vi "provide_OME_data.vi"(6 "image ID":string, 8 "error in (no error)":errorcluster, 9 "structuredAttribute string in":string, 10 "OME element in":refnum<class "XMLElement.lvclass">, 11 "GenericDataCollection in":refnum<class "GenericDataCollection.lvclass">) -> (0 "error out":errorcluster, 1 "structuredAttribute string out":string, 2 "OME element out":refnum<class "XMLElement.lvclass">, 3 "GenericDataCollection out":refnum<class "GenericDataCollection.lvclass">)   [LabVIEW 2010, in "GenericDataCollection.lvclass"]
uses:
  GenericDataCollection.lvclass
  common/classes/XMLElement/XMLElement/XMLElement.lvclass
  ImagingMode/GenericImagingMode/GenericImagingMode/GenericImagingMode.lvclass
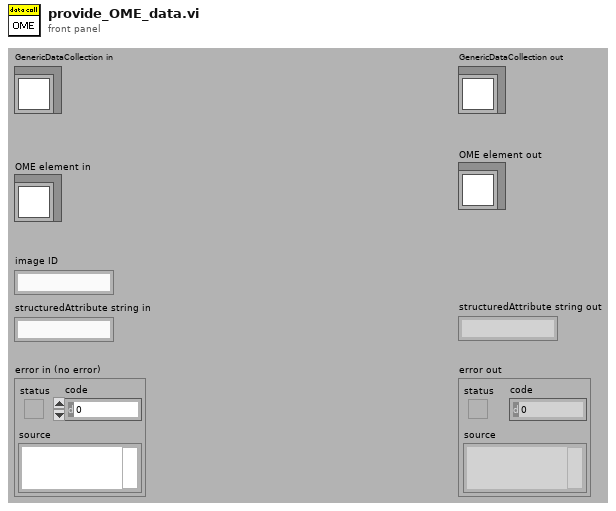
[diagram p1: front panel]
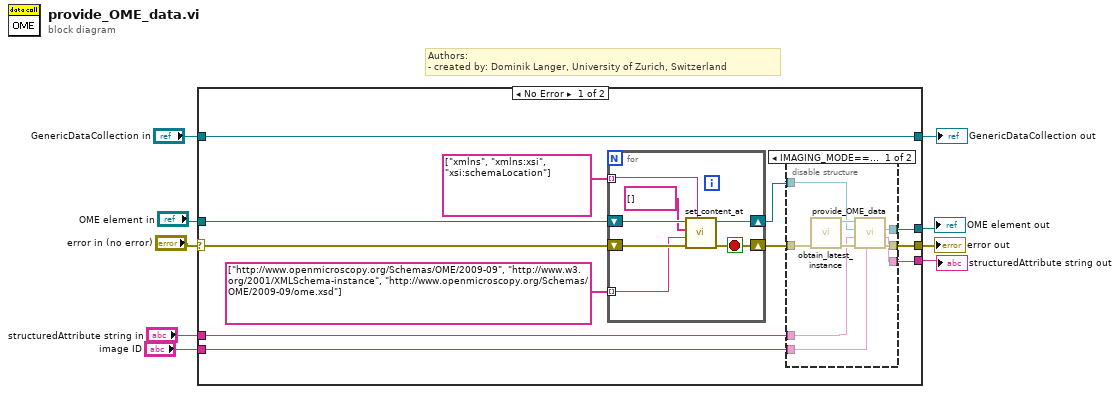
[diagram p0: block diagram]
diagram:
  # "Authors: \n- created by: Dominik Langer, University of Zurich, Switzerland"
  n1 = case shown="No Error" "error in (no error)" {
    selector: "error in (no error)" -> [w20 w44]
    tunnel: [w16 w44] -> w9
    tunnel: [w21 w43] -> w8
    tunnel: "GenericDataCollection in" -> [w21 w43]
    tunnel: [w15 w42] -> w3
    tunnel: "OME element in" -> [w19 w42]
    tunnel: "image ID" -> [w12 _]
    tunnel: "structuredAttribute string in" -> [w11 w41]
    tunnel: [w10 w41] -> w1
    frame No Error {
      n2 = for {
        shift-right: [w34] -> w14
        shift-left: w20 -> [w40]
        shift-right: [w38] -> w13
        shift-left: w19 -> [w39]
        tunnel: string[] ["xmlns", "xmlns:xsi", "xsi:schemaLocation"] ("key array") -> [w37] mode=indexing
        tunnel: string[] ["http://www.openmicroscopy.org/Schemas/OME/2009-09", "http://www.w3.org/2001/XMLSchema-instance", "http://www.openmicroscopy.org/Schemas/OME/2009-09/ome.xsd"] -> [w36] mode=indexing
        stop <- w34 stop-if-true
        n3 = call "set_content_at.vi"("attribute name"=w37, "error in (no error)"=w40, "content"=w36, "key chain"=string[] [], "Element in"=w39) -> ("error out"=w34:errorcluster, "Element out"=w38:refnum<class "XMLElement.lvclass">)  [unwired: 5 in]
      }
      n4 = disable-structure shown="IMAGING_MODE==1" {
        disable-tunnel: w14 -> [w30 w33]
        disable-tunnel: w13 -> [w27 w32]
        disable-tunnel: w12 -> [w24 _]
        disable-tunnel: [w26 w33] -> w16
        disable-tunnel: [w25 w32] -> w15
        disable-tunnel: w11 -> [w23 w31]
        disable-tunnel: [w22 w31] -> w10
        frame condition #0 {
          n5 = call "obtain_latest_instance.vi"("error in (no error)"=w30) -> ("error out"=w29:errorcluster, "GenericScanMode out"=w28:refnum<class "GenericImagingMode.lvclass">)  [unwired: 9 in]
          n6 = call-dynamic "provide_OME_data.vi"("image ID"=w24, "error in (no error)"=w29, "structuredAttribute string in"=w23, "OME element in"=w27, "GenericPlugin in"=w28) -> ("error out"=w26:errorcluster, "structuredAttribute string out"=w22:string, "OME element out"=w25:refnum<class "XMLElement.lvclass">)  [unwired: 3 in, 1 out]
        }
        frame condition #1 (active) {
        }
      }
    }
    frame Error {
    }
  }
  "error out" <- w9
  "GenericDataCollection out" <- w8
  "OME element out" <- w3
  "structuredAttribute string out" <- w1
